vi "myRIO_BRig_RT_dataCurrent_init.vi"() -> (3 "output_dataCurrent":u16[](array[numeric]))   [LabVIEW 2014]
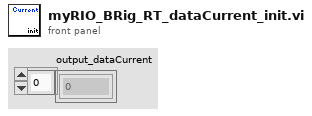
[diagram p1: front panel]
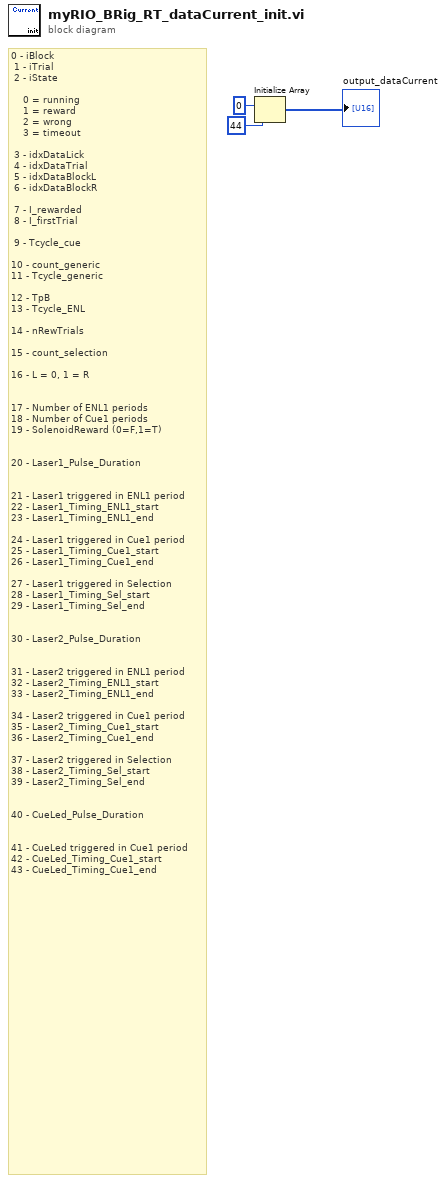
[diagram p0: block diagram]
diagram:
  # "0 - iBlock\n 1 - iTrial\n 2 - iState\n\n    0 = running\n    1 = reward\n    2 = wrong\n    3 = timeout\n\n 3 - idxDataLick\n 4 - idxDataTrial\n 5 - idxDataBlockL\n 6 - idxDataBlockR\n\n 7 - I_rewarded\n 8 - I_firstTrial\n\n 9 - Tcycle_cue\n\n10 - count_generic\n11 - Tcycle_generic\n\n12 - TpB\n13 - Tcycle_ENL\n\n14 - nRewTrials\n\n15 - count_selection\n\n16 - L = 0, 1 = R\n\n\n17 - Number of ENL1 periods\n18 - Number of Cue1 periods\n19 - SolenoidReward (0=F,1=T)\n\n\n20 - Laser1_Pulse_Duration\n\n\n21 - Laser1 triggered in ENL1 period\n22 - Laser1_Timing_ENL1_start\n23 - Laser1_Timing_ENL1_end\n\n24 - Laser1 triggered in Cue1 period\n25 - Laser1_Timing_Cue1_start\n26 - Laser1_Timing_Cue1_end\n\n27 - Laser1 triggered in Selection\n28 - Laser1_Timing_Sel_start\n29 - Laser1_Timing_Sel_end\n\n\n30 - Laser2_Pulse_Duration\n\n\n31 - Laser2 triggered in ENL1 period\n32 - Laser2_Timing_ENL1_start\n33 - Laser2_Timing_ENL1_end\n\n34 - Laser2 triggered in Cue1 period\n35 - Laser2_Timing_Cue1_start\n36 - Laser2_Timing_Cue1_end\n\n37 - Laser2 triggered in Selection\n38 - Laser2_Timing_Sel_start\n39 - Laser2_Timing_Sel_end\n\n\n40 - CueLed_Pulse_Duration\n\n\n41 - CueLed triggered in Cue1 period\n42 - CueLed_Timing_Cue1_start\n43 - CueLed_Timing_Cue1_end"
  n1 = Initialize Array(u16 0 ("element"), 44 ("dimension size")) -> (→"output_dataCurrent":u16[])
